vi "Get all frames from buffer.vi"(8 "error in (no error)":errorcluster, 11 "uCAN in":refnum<class "uCAN.lvclass">) -> (0 "error out":errorcluster, 2 "Received Frames Array":T1[](array[typedef]) {"Data" format="%.0x"}, 3 "uCAN out":refnum<class "uCAN.lvclass">)   [LabVIEW 2021, in "uCanDriver.lvlib" / "uCAN.lvclass"]
uses:
  uCAN.lvclass
  typedefs/frame.ctl
  uCAN.lvclass/uCAN.ctl
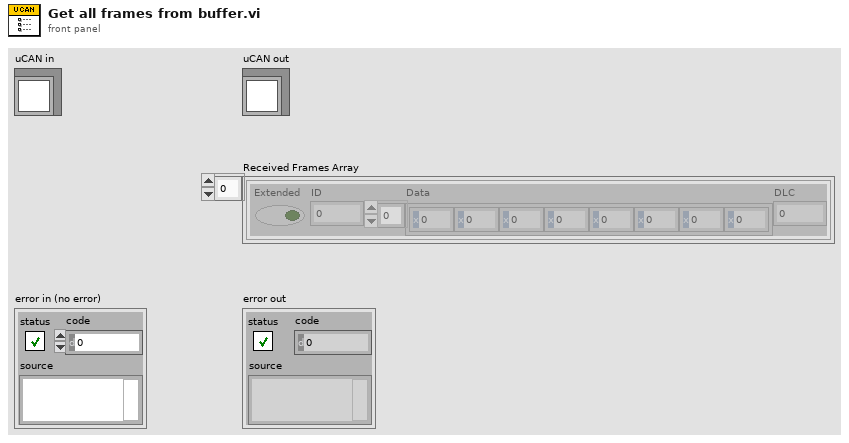
[diagram p1: front panel]
types:
  T1 = typedef "uCanDriver.lvlib/uCAN.lvclass/frame.ctl" = cluster{"Extended":bool, "ID":u32, "Data":u8[], "DLC":u8}
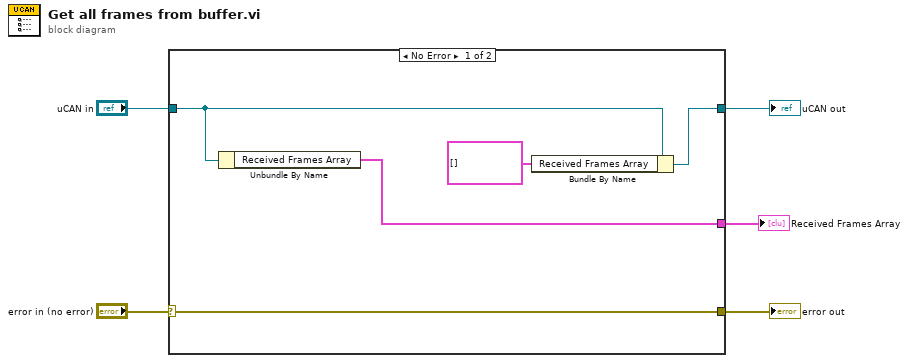
[diagram p0: block diagram]
diagram:
  n1 = case shown="No Error" "error in (no error)" {
    selector: "error in (no error)" -> [w10 w12]
    tunnel: [w10 w12] -> w4
    tunnel: [w8 w11] -> w2
    tunnel: "uCAN in" -> [w9 w11]
    tunnel: [w6 _] -> w1
    frame No Error {
      n2 = Unbundle By Name(w9) -> ("Received Frames Array"=w6:T1[])
      n3 = Bundle By Name(cluster=w9, "Received Frames Array"=T1[] []) -> (w8:refnum<class "uCAN.lvclass">)
    }
    frame Error {
    }
  }
  "error out" <- w4
  "uCAN out" <- w2
  "Received Frames Array" <- w1
